vi "test TCX read (installed 71).vi"() -> ()   [LabVIEW 2011] (continued)
xmlns=\"http://www.garmin.com/xmlschemas/ActivityExtension/v2\"><Watts>107</Watts></TPX></Extensions></Trackpoint><Trackpoint><Time>2008-03-03T14:04:57Z</Time><Position><LatitudeDegrees>35.860918</LatitudeDegrees><LongitudeDegrees>-78.895742</LongitudeDegrees></Position><AltitudeMeters>90.021</AltitudeMeters><DistanceMeters>8842.457</DistanceMeters><Cadence>0</Cadence></Trackpoint><Trackpoint><Time>2008-03-03T14:04:58Z</Time><Position><LatitudeDegrees>35.860915</LatitudeDegrees><LongitudeDegrees>-78.895606</LongitudeDegrees></Position><AltitudeMeters>90.021</AltitudeMeters><DistanceMeters>8854.741</DistanceMeters><Cadence>0</Cadence></Trackpoint><Trackpoint><Time>2008-03-03T14:04:59Z</Time><Position><LatitudeDegrees>35.860920</LatitudeDegrees><LongitudeDegrees>-78.895468</LongitudeDegrees></Position><AltitudeMeters>89.059</AltitudeMeters><DistanceMeters>8867.175</DistanceMeters><Cadence>0</Cadence></Trackpoint><Trackpoint><Time>2008-03-03T14:05:00Z</Time><Position><LatitudeDegrees>35.860930</LatitudeDegrees><LongitudeDegrees>-78.895327</LongitudeDegrees></Position><AltitudeMeters>87.617</AltitudeMeters><DistanceMeters>8879.941</DistanceMeters><Cadence>0</Cadence></Trackpoint><Trackpoint><Time>2008-03-03T14:05:01Z</Time><Position><LatitudeDegrees>35.860938</LatitudeDegrees><LongitudeDegrees>-78.895183</LongitudeDegrees></Position><AltitudeMeters>87.137</AltitudeMeters><DistanceMeters>8893.053</DistanceMeters><Cadence>0</Cadence></Trackpoint><Trackpoint><Time>2008-03-03T14:05:02Z</Time><Position><LatitudeDegrees>35.860939</LatitudeDegrees><LongitudeDegrees>-78.895036</LongitudeDegrees></Position><AltitudeMeters>86.656</AltitudeMeters><DistanceMeters>8906.286</DistanceMeters><Cadence>0</Cadence></Trackpoint><Trackpoint><Time>2008-03-03T14:05:03Z</Time><Position><LatitudeDegrees>35.860942</LatitudeDegrees><LongitudeDegrees>-78.894890</LongitudeDegrees></Position><AltitudeMeters>85.695</AltitudeMeters><DistanceMeters>8919.586</DistanceMeters><Cadence>0</Cadence></Trackpoint><Trackpoint><Time>2008-03-03T14:05:04Z</Time><Position><LatitudeDegrees>35.860938</LatitudeDegrees><LongitudeDegrees>-78.894740</LongitudeDegrees></Position><AltitudeMeters>85.214</AltitudeMeters><DistanceMeters>8933.086</DistanceMeters><Cadence>0</Cadence></Trackpoint><Trackpoint><Time>2008-03-03T14:05:05Z</Time><Position><LatitudeDegrees>35.860924</LatitudeDegrees><LongitudeDegrees>-78.894592</LongitudeDegrees></Position><AltitudeMeters>84.253</AltitudeMeters><DistanceMeters>8946.535</DistanceMeters><Cadence>0</Cadence></Trackpoint><Trackpoint><Time>2008-03-03T14:05:06Z</Time><Position><LatitudeDegrees>35.860898</LatitudeDegrees><LongitudeDegrees>-78.894446</LongitudeDegrees></Position><AltitudeMeters>83.291</AltitudeMeters><DistanceMeters>8959.948</DistanceMeters><Cadence>0</Cadence></Trackpoint><Trackpoint><Time>2008-03-03T14:05:07Z</Time><Position><LatitudeDegrees>35.860875</LatitudeDegrees><LongitudeDegrees>-78.894304</LongitudeDegrees></Position><AltitudeMeters>83.772</AltitudeMeters><DistanceMeters>8973.048</DistanceMeters><Cadence>0</Cadence></Trackpoint><Trackpoint><Time>2008-03-03T14:05:08Z</Time><Position><LatitudeDegrees>35.860851</LatitudeDegrees><LongitudeDegrees>-78.894163</LongitudeDegrees></Position><AltitudeMeters>82.811</AltitudeMeters><DistanceMeters>8985.948</DistanceMeters><Cadence>0</Cadence></Trackpoint><Trackpoint><Time>2008-03-03T14:05:09Z</Time><Position><LatitudeDegrees>35.860831</LatitudeDegrees><LongitudeDegrees>-78.894026</LongitudeDegrees></Position><AltitudeMeters>82.330</AltitudeMeters><DistanceMeters>8998.589</DistanceMeters><Cadence>0</Cadence></Trackpoint><Trackpoint><Time>2008-03-03T14:05:10Z</Time><Position><LatitudeDegrees>35.860809</LatitudeDegrees><LongitudeDegrees>-78.893890</LongitudeDegrees></Position><AltitudeMeters>81.849</AltitudeMeters><DistanceMeters>9011.048</DistanceMeters><Cadence>4</Cadence><Extensions><TPX xmlns=\"http://www.garmin.com/xmlschemas/ActivityExtension/v2\"><Watts>0</Watts></TPX></Extensions></Trackpoint><Trackpoint><Time>2008-03-03T14:05:11Z</Time><Position><LatitudeDegrees>35.860788</LatitudeDegrees><LongitudeDegrees>-78.893758</LongitudeDegrees></Position><AltitudeMeters>81.849</AltitudeMeters><DistanceMeters>9023.194</DistanceMeters><Cadence>4</Cadence><Extensions><TPX xmlns=\"http://www.garmin.com/xmlschemas/ActivityExtension/v2\"><Watts>0</Watts></TPX></Extensions></Trackpoint><Trackpoint><Time>2008-03-03T14:05:12Z</Time><Position><LatitudeDegrees>35.860769</LatitudeDegrees><LongitudeDegrees>-78.893628</LongitudeDegrees></Position><AltitudeMeters>81.369</AltitudeMeters><DistanceMeters>9035.092</DistanceMeters><Cadence>71</Cadence><Extensions><TPX xmlns=\"http://www.garmin.com/xmlschemas/ActivityExtension/v2\"><Watts>90</Watts></TPX></Extensions></Trackpoint><Trackpoint><Time>2008-03-03T14:05:13Z</Time><Position><LatitudeDegrees>35.860753</LatitudeDegrees><LongitudeDegrees>-78.893502</LongitudeDegrees></Position><AltitudeMeters>81.849</AltitudeMeters><DistanceMeters>9046.647</DistanceMeters><Cadence>84</Cadence><Extensions><TPX xmlns=\"http://www.garmin.com/xmlschemas/ActivityExtension/v2\"><Watts>145</Watts></TPX></Extensions></Trackpoint><Trackpoint><Time>2008-03-03T14:05:14Z</Time><Position><LatitudeDegrees>35.860738</LatitudeDegrees><LongitudeDegrees>-78.893381</LongitudeDegrees></Position><AltitudeMeters>81.849</AltitudeMeters><DistanceMeters>9057.588</DistanceMeters><Cadence>81</Cadence><Extensions><TPX xmlns=\"http://www.garmin.com/xmlschemas/ActivityExtension/v2\"><Watts>197</Watts></TPX></Extensions></Trackpoint><Trackpoint><Time>2008-03-03T14:05:15Z</Time><Position><LatitudeDegrees>35.860725</LatitudeDegrees><LongitudeDegrees>-78.893268</LongitudeDegrees></Position><AltitudeMeters>82.811</AltitudeMeters><DistanceMeters>9067.873</DistanceMeters><Cadence>80</Cadence><Extensions><TPX xmlns=\"http://www.garmin.com/xmlschemas/ActivityExtension/v2\"><Watts>211</Watts></TPX></Extensions></Trackpoint><Trackpoint><Time>2008-03-03T14:05:16Z</Time><Position><LatitudeDegrees>35.860714</LatitudeDegrees><LongitudeDegrees>-78.893164</LongitudeDegrees></Position><AltitudeMeters>83.291</AltitudeMeters><DistanceMeters>9077.331</DistanceMeters><Cadence>78</Cadence><Extensions><TPX xmlns=\"http://www.garmin.com/xmlschemas/ActivityExtension/v2\"><Watts>233</Watts></TPX></Extensions></Trackpoint><Trackpoint><Time>2008-03-03T14:05:17Z</Time><Position><LatitudeDegrees>35.860703</LatitudeDegrees><LongitudeDegrees>-78.893065</LongitudeDegrees></Position><AltitudeMeters>84.253</AltitudeMeters><DistanceMeters>9086.308</DistanceMeters><Cadence>73</Cadence><Extensions><TPX xmlns=\"http://www.garmin.com/xmlschemas/ActivityExtension/v2\"><Watts>281</Watts></TPX></Extensions></Trackpoint><Trackpoint><Time>2008-03-03T14:05:18Z</Time><Position><LatitudeDegrees>35.860691</LatitudeDegrees><LongitudeDegrees>-78.892970</LongitudeDegrees></Position><AltitudeMeters>84.253</AltitudeMeters><DistanceMeters>9095.026</DistanceMeters><Cadence>73</Cadence><Extensions><TPX xmlns=\"http://www.garmin.com/xmlschemas/ActivityExtension/v2\"><Watts>281</Watts></TPX></Extensions></Trackpoint><Trackpoint><Time>2008-03-03T14:05:19Z</Time><Position><LatitudeDegrees>35.860678</LatitudeDegrees><LongitudeDegrees>-78.892875</LongitudeDegrees></Position><AltitudeMeters>84.733</AltitudeMeters><DistanceMeters>9103.671</DistanceMeters><Cadence>72</Cadence><Extensions><TPX xmlns=\"http://www.garmin.com/xmlschemas/ActivityExtension/v2\"><Watts>458</Watts></TPX></Extensions></Trackpoint><Trackpoint><Time>2008-03-03T14:05:20Z</Time><Position><LatitudeDegrees>35.860666</LatitudeDegrees><LongitudeDegrees>-78.892780</LongitudeDegrees></Position><AltitudeMeters>84.733</AltitudeMeters><DistanceMeters>9112.350</DistanceMeters><Cadence>72</Cadence><Extensions><TPX xmlns=\"http://www.garmin.com/xmlschemas/ActivityExtension/v2\"><Watts>588</Watts></TPX></Extensions></Trackpoint><Trackpoint><Time>2008-03-03T14:05:21Z</Time><Position><LatitudeDegrees>35.860655</LatitudeDegrees><LongitudeDegrees>-78.892685</LongitudeDegrees></Position><AltitudeMeters>85.214</AltitudeMeters><DistanceMeters>9121.041</DistanceMeters><Cadence>72</Cadence><Extensions><TPX xmlns=\"http://www.garmin.com/xmlschemas/ActivityExtension/v2\"><Watts>591</Watts></TPX></Extensions></Trackpoint><Trackpoint><Time>2008-03-03T14:05:22Z</Time><Position><LatitudeDegrees>35.860642</LatitudeDegrees><LongitudeDegrees>-78.892589</LongitudeDegrees></Position><AltitudeMeters>85.214</AltitudeMeters><DistanceMeters>9129.810</DistanceMeters><Cadence>72</Cadence><Extensions><TPX xmlns=\"http://www.garmin.com/xmlschemas/ActivityExtension/v2\"><Watts>493</Watts></TPX></Extensions></Trackpoint><Trackpoint><Time>2008-03-03T14:05:23Z</Time><Position><LatitudeDegrees>35.860628</LatitudeDegrees><LongitudeDegrees>-78.892493</LongitudeDegrees></Position><AltitudeMeters>85.695</AltitudeMeters><DistanceMeters>9138.619</DistanceMeters><Cadence>72</Cadence><Extensions><TPX xmlns=\"http://www.garmin.com/xmlschemas/ActivityExtension/v2\"><Watts>472</Watts></TPX></Extensions></Trackpoint><Trackpoint><Time>2008-03-03T14:05:24Z</Time><Position><LatitudeDegrees>35.860618</LatitudeDegrees><LongitudeDegrees>-78.892396</LongitudeDegrees></Position><AltitudeMeters>86.175</AltitudeMeters><DistanceMeters>9147.436</DistanceMeters><Cadence>73</Cadence><Extensions><TPX xmlns=\"http://www.garmin.com/xmlschemas/ActivityExtension/v2\"><Watts>438</Watts></TPX></Extensions></Trackpoint><Trackpoint><Time>2008-03-03T14:05:25Z</Time><Position><LatitudeDegrees>35.860608</LatitudeDegrees><LongitudeDegrees>-78.892296</LongitudeDegrees></Position><AltitudeMeters>85.695</AltitudeMeters><DistanceMeters>9156.547</DistanceMeters><Cadence>74</Cadence><Extensions><TPX xmlns=\"http://www.garmin.com/xmlschemas/ActivityExtension/v2\"><Watts>433</Watts></TPX></Extensions></Trackpoint><Trackpoint><Time>2008-03-03T14:05:26Z</Time><Position><LatitudeDegrees>35.860601</LatitudeDegrees><LongitudeDegrees>-78.892192</LongitudeDegrees></Position><AltitudeMeters>86.175</AltitudeMeters><DistanceMeters>9165.991</DistanceMeters><Cadence>76</Cadence><Extensions><TPX xmlns=\"http://www.garmin.com/xmlschemas/ActivityExtension/v2\"><Watts>430</Watts></TPX></Extensions></Trackpoint><Trackpoint><Time>2008-03-03T14:05:27Z</Time><Position><LatitudeDegrees>35.860591</LatitudeDegrees><LongitudeDegrees>-78.892087</LongitudeDegrees></Position><AltitudeMeters>86.656</AltitudeMeters><DistanceMeters>9175.522</DistanceMeters><Cadence>80</Cadence><Extensions><TPX xmlns=\"http://www.garmin.com/xmlschemas/ActivityExtension/v2\"><Watts>528</Watts></TPX></Extensions></Trackpoint><Trackpoint><Time>2008-03-03T14:05:28Z</Time><Position><LatitudeDegrees>35.860585</LatitudeDegrees><LongitudeDegrees>-78.891979</LongitudeDegrees></Position><AltitudeMeters>86.175</AltitudeMeters><DistanceMeters>9185.361</DistanceMeters><Cadence>81</Cadence><Extensions><TPX xmlns=\"http://www.garmin.com/xmlschemas/ActivityExtension/v2\"><Watts>536</Watts></TPX></Extensions></Trackpoint><Trackpoint><Time>2008-03-03T14:05:29Z</Time><Position><LatitudeDegrees>35.860574</LatitudeDegrees><LongitudeDegrees>-78.891869</LongitudeDegrees></Position><AltitudeMeters>87.137</AltitudeMeters><DistanceMeters>9195.392</DistanceMeters><Cadence>82</Cadence><Extensions><TPX xmlns=\"http://www.garmin.com/xmlschemas/ActivityExtension/v2\"><Watts>542</Watts></TPX></Extensions></Trackpoint><Trackpoint><Time>2008-03-03T14:05:30Z</Time><Position><LatitudeDegrees>35.860564</LatitudeDegrees><LongitudeDegrees>-78.891759</LongitudeDegrees></Position><AltitudeMeters>87.137</AltitudeMeters><DistanceMeters>9205.390</DistanceMeters><Cadence>82</Cadence><Extensions><TPX xmlns=\"http://www.garmin.com/xmlschemas/ActivityExtension/v2\"><Watts>523</Watts></TPX></Extensions></Trackpoint><Trackpoint><Time>2008-03-03T14:05:31Z</Time><Position><LatitudeDegrees>35.860551</LatitudeDegrees><LongitudeDegrees>-78.891649</LongitudeDegrees></Position><AltitudeMeters>87.617</AltitudeMeters><DistanceMeters>9215.414</DistanceMeters><Cadence>86</Cadence><Extensions><TPX xmlns=\"http://www.garmin.com/xmlschemas/ActivityExtension/v2\"><Watts>515</Watts></TPX></Extensions></Trackpoint><Trackpoint><Time>2008-03-03T14:05:32Z</Time><Position><LatitudeDegrees>35.860540</LatitudeDegrees><LongitudeDegrees>-78.891537</LongitudeDegrees></Position><AltitudeMeters>87.617</AltitudeMeters><DistanceMeters>9225.561</DistanceMeters><Cadence>82</Cadence><Extensions><TPX xmlns=\"http://www.garmin.com/xmlschemas/ActivityExtension/v2\"><Watts>495</Watts></TPX></Extensions></Trackpoint><Trackpoint><Time>2008-03-03T14:05:33Z</Time><Position><LatitudeDegrees>35.860528</LatitudeDegrees><LongitudeDegrees>-78.891428</LongitudeDegrees></Position><AltitudeMeters>87.617</AltitudeMeters><DistanceMeters>9235.504</DistanceMeters><Cadence>80</Cadence><Extensions><TPX xmlns=\"http://www.garmin.com/xmlschemas/ActivityExtension/v2\"><Watts>168</Watts></TPX></Extensions></Trackpoint><Trackpoint><Time>2008-03-03T14:05:34Z</Time><Position><LatitudeDegrees>35.860516</LatitudeDegrees><LongitudeDegrees>-78.891323</LongitudeDegrees></Position><AltitudeMeters>87.617</AltitudeMeters><DistanceMeters>9245.120</DistanceMeters><Cadence>78</Cadence><Extensions><TPX xmlns=\"http://www.garmin.com/xmlschemas/ActivityExtension/v2\"><Watts>157</Watts></TPX></Extensions></Trackpoint><Trackpoint><Time>2008-03-03T14:05:35Z</Time><Position><LatitudeDegrees>35.860506</LatitudeDegrees><LongitudeDegrees>-78.891219</LongitudeDegrees></Position><AltitudeMeters>87.617</AltitudeMeters><DistanceMeters>9254.466</DistanceMeters><Cadence>76</Cadence><Extensions><TPX xmlns=\"http://www.garmin.com/xmlschemas/ActivityExtension/v2\"><Watts>146</Watts></TPX></Extensions></Trackpoint><Trackpoint><Time>2008-03-03T14:05:36Z</Time><Position><LatitudeDegrees>35.860495</LatitudeDegrees><LongitudeDegrees>-78.891119</LongitudeDegrees></Position><AltitudeMeters>87.617</AltitudeMeters><DistanceMeters>9263.595</DistanceMeters><Cadence>75</Cadence><Extensions><TPX xmlns=\"http://www.garmin.com/xmlschemas/ActivityExtension/v2\"><Watts>141</Watts></TPX></Extensions></Trackpoint><Trackpoint><Time>2008-03-03T14:05:37Z</Time><Position><LatitudeDegrees>35.860483</LatitudeDegrees><LongitudeDegrees>-78.891021</LongitudeDegrees></Position><AltitudeMeters>87.617</AltitudeMeters><DistanceMeters>9272.575</DistanceMeters><Cadence>73</Cadence><Extensions><TPX xmlns=\"http://www.garmin.com/xmlschemas/ActivityExtension/v2\"><Watts>139</Watts></TPX></Extensions></Trackpoint><Trackpoint><Time>2008-03-03T14:05:38Z</Time><Position><LatitudeDegrees>35.860470</LatitudeDegrees><LongitudeDegrees>-78.890924</LongitudeDegrees></Position><AltitudeMeters>87.617</AltitudeMeters><DistanceMeters>9281.458</DistanceMeters><Cadence>72</Cadence><Extensions><TPX xmlns=\"http://www.garmin.com/xmlschemas/ActivityExtension/v2\"><Watts>141</Watts></TPX></Extensions></Trackpoint><Trackpoint><Time>2008-03-03T14:05:39Z</Time><Position><LatitudeDegrees>35.860457</LatitudeDegrees><LongitudeDegrees>-78.890829</LongitudeDegrees></Position><AltitudeMeters>88.098</AltitudeMeters><DistanceMeters>9290.096</DistanceMeters><Cadence>71</Cadence><Extensions><TPX xmlns=\"http://www.garmin.com/xmlschemas/ActivityExtension/v2\"><Watts>141</Watts></TPX></Extensions></Trackpoint><Trackpoint><Time>2008-03-03T14:05:40Z</Time><Position><LatitudeDegrees>35.860444</LatitudeDegrees><LongitudeDegrees>-78.890736</LongitudeDegrees></Position><AltitudeMeters>88.098</AltitudeMeters><DistanceMeters>9298.659</DistanceMeters><Cadence>71</Cadence><Extensions><TPX xmlns=\"http://www.garmin.com/xmlschemas/ActivityExtension/v2\"><Watts>140</Watts></TPX></Extensions></Trackpoint><Trackpoint><Time>2008-03-03T14:05:41Z</Time><Position><LatitudeDegrees>35.860431</LatitudeDegrees><LongitudeDegrees>-78.890644</LongitudeDegrees></Position><AltitudeMeters>88.098</AltitudeMeters><DistanceMeters>9307.081</DistanceMeters><Cadence>70</Cadence><Extensions><TPX xmlns=\"http://www.garmin.com/xmlschemas/ActivityExtension/v2\"><Watts>150</Watts></TPX></Extensions></Trackpoint><Trackpoint><Time>2008-03-03T14:05:42Z</Time><Position><LatitudeDegrees>35.860420</LatitudeDegrees><LongitudeDegrees>-78.890553</LongitudeDegrees></Position><AltitudeMeters>88.098</AltitudeMeters><DistanceMeters>9315.363</DistanceMeters><Cadence>74</Cadence><Extensions><TPX xmlns=\"http://www.garmin.com/xmlschemas/ActivityExtension/v2\"><Watts>141</Watts></TPX></Extensions></Trackpoint><Trackpoint><Time>2008-03-03T14:05:43Z</Time><Position><LatitudeDegrees>35.860407</LatitudeDegrees><LongitudeDegrees>-78.890463</LongitudeDegrees></Position><AltitudeMeters>88.579</AltitudeMeters><DistanceMeters>9323.592</DistanceMeters><Cadence>76</Cadence><Extensions><TPX xmlns=\"http://www.garmin.com/xmlschemas/ActivityExtension/v2\"><Watts>133</Watts></TPX></Extensions></Trackpoint><Trackpoint><Time>2008-03-03T14:05:44Z</Time><Position><LatitudeDegrees>35.860393</LatitudeDegrees><LongitudeDegrees>-78.890375</LongitudeDegrees></Position><AltitudeMeters>88.579</AltitudeMeters><DistanceMeters>9331.684</DistanceMeters><Cadence>75</Cadence><Extensions><TPX xmlns=\"http://www.garmin.com/xmlschemas/ActivityExtension/v2\"><Watts>171</Watts></TPX></Extensions></Trackpoint><Trackpoint><Time>2008-03-03T14:05:45Z</Time><Position><LatitudeDegrees>35.860381</LatitudeDegrees><LongitudeDegrees>-78.890287</LongitudeDegrees></Position><AltitudeMeters>89.059</AltitudeMeters><DistanceMeters>9339.685</DistanceMeters><Cadence>75</Cadence><Extensions><TPX xmlns=\"http://www.garmin.com/xmlschemas/ActivityExtension/v2\"><Watts>207</Watts></TPX></Extensions></Trackpoint><Trackpoint><Time>2008-03-03T14:05:46Z</Time><Position><LatitudeDegrees>35.860372</LatitudeDegrees><LongitudeDegrees>-78.890200</LongitudeDegrees></Position><AltitudeMeters>88.579</AltitudeMeters><DistanceMeters>9347.658</DistanceMeters><Cadence>74</Cadence><Extensions><TPX xmlns=\"http://www.garmin.com/xmlschemas/ActivityExtension/v2\"><Watts>227</Watts></TPX></Extensions></Trackpoint><Trackpoint><Time>2008-03-03T14:05:47Z</Time><Position><LatitudeDegrees>35.860362</LatitudeDegrees><LongitudeDegrees>-78.890113</LongitudeDegrees></Position><AltitudeMeters>89.059</AltitudeMeters><DistanceMeters>9355.555</DistanceMeters><Cadence>73</Cadence><Extensions><TPX xmlns=\"http://www.garmin.com/xmlschemas/ActivityExtension/v2\"><Watts>228</Watts></TPX></Extensions></Trackpoint><Trackpoint><Time>2008-03-03T14:05:48Z</Time><Position><LatitudeDegrees>35.860352</LatitudeDegrees><LongitudeDegrees>-78.890027</LongitudeDegrees></Position><AltitudeMeters>89.540</AltitudeMeters><DistanceMeters>9363.416</DistanceMeters><Cadence>73</Cadence><Extensions><TPX xmlns=\"http://www.garmin.com/xmlschemas/ActivityExtension/v2\"><Watts>231</Watts></TPX></Extensions></Trackpoint><Trackpoint><Time>2008-03-03T14:05:49Z</Time><Position><LatitudeDegrees>35.860343</LatitudeDegrees><LongitudeDegrees>-78.889942</LongitudeDegrees></Position><AltitudeMeters>89.540</AltitudeMeters><DistanceMeters>9371.137</DistanceMeters><Cadence>72</Cadence><Extensions><TPX xmlns=\"http://www.garmin.com/xmlschemas/ActivityExtension/v2\"><Watts>246</Watts></TPX></Extensions></Trackpoint><Trackpoint><Time>2008-03-03T14:05:50Z</Time><Position><LatitudeDegrees>35.860334</LatitudeDegrees><LongitudeDegrees>-78.889859</LongitudeDegrees></Position><AltitudeMeters>90.021</AltitudeMeters><DistanceMeters>9378.760</DistanceMeters><Cadence>72</Cadence><Extensions><TPX xmlns=\"http://www.garmin.com/xmlschemas/ActivityExtension/v2\"><Watts>246</Watts></TPX></Extensions></Trackpoint><Trackpoint><Time>2008-03-03T14:05:51Z</Time><Position><LatitudeDegrees>35.860323</LatitudeDegrees><LongitudeDegrees>-78.889776</LongitudeDegrees></Position><AltitudeMeters>90.021</AltitudeMeters><DistanceMeters>9386.328</DistanceMeters><Cadence>70</Cadence><Extensions><TPX xmlns=\"http://www.garmin.com/xmlschemas/ActivityExtension/v2\"><Watts>306</Watts></TPX></Extensions></Trackpoint><Trackpoint><Time>2008-03-03T14:05:52Z</Time><Position><LatitudeDegrees>35.860313</LatitudeDegrees><LongitudeDegrees>-78.889694</LongitudeDegrees></Position><AltitudeMeters>90.501</AltitudeMeters><DistanceMeters>9393.784</DistanceMeters><Cadence>70</Cadence><Extensions><TPX xmlns=\"http://www.garmin.com/xmlschemas/ActivityExtension/v2\"><Watts>305</Watts></TPX></Extensions></Trackpoint><Trackpoint><Time>2008-03-03T14:05:53Z</Time><Position><LatitudeDegrees>35.860303</LatitudeDegrees><LongitudeDegrees>-78.889613</LongitudeDegrees></Position><AltitudeMeters>90.982</AltitudeMeters><DistanceMeters>9401.264</DistanceMeters><Cadence>69</Cadence><Extensions><TPX xmlns=\"http://www.garmin.com/xmlschemas/ActivityExtension/v2\"><Watts>334</Watts></TPX></Extensions></Trackpoint><Trackpoint><Time>2008-03-03T14:05:54Z</Time><Position><LatitudeDegrees>35.860294</LatitudeDegrees><LongitudeDegrees>-78.889530</LongitudeDegrees></Position><AltitudeMeters>91.463</AltitudeMeters><DistanceMeters>9408.714</DistanceMeters><Cadence>70</Cadence><Extensions><TPX xmlns=\"http://www.garmin.com/xmlschemas/ActivityExtension/v2\"><Watts>368</Watts></TPX></Extensions></Trackpoint><Trackpoint><Time>2008-03-03T14:05:55Z</Time><Position><LatitudeDegrees>35.860285</LatitudeDegrees><LongitudeDegrees>-78.889448</LongitudeDegrees></Position><AltitudeMeters>91.463</AltitudeMeters><DistanceMeters>9416.229</DistanceMeters><Cadence>70</Cadence><Extensions><TPX xmlns=\"http://www.garmin.com/xmlschemas/ActivityExtension/v2\"><Watts>382</Watts></TPX></Extensions></Trackpoint><Trackpoint><Time>2008-03-03T14:05:56Z</Time><Position><LatitudeDegrees>35.860275</LatitudeDegrees><LongitudeDegrees>-78.889366</LongitudeDegrees></Position><AltitudeMeters>91.463</AltitudeMeters><DistanceMeters>9423.748</DistanceMeters><Cadence>70</Cadence><Extensions><TPX xmlns=\"http://www.garmin.com/xmlschemas/ActivityExtension/v2\"><Watts>382</Watts></TPX></Extensions></Trackpoint><Trackpoint><Time>2008-03-03T14:05:57Z</Time><Position><LatitudeDegrees>35.860264</LatitudeDegrees><LongitudeDegrees>-78.889285</LongitudeDegrees></Position><AltitudeMeters>91.943</AltitudeMeters><DistanceMeters>9431.158</DistanceMeters><Cadence>70</Cadence><Extensions><TPX xmlns=\"http://www.garmin.com/xmlschemas/ActivityExtension/v2\"><Watts>383</Watts></TPX></Extensions></Trackpoint><Trackpoint><Time>2008-03-03T14:05:58Z</Time><Position><LatitudeDegrees>35.860254</LatitudeDegrees><LongitudeDegrees>-78.889204</LongitudeDegrees></Position><AltitudeMeters>92.424</AltitudeMeters><DistanceMeters>9438.506</DistanceMeters><Cadence>68</Cadence><Extensions><TPX xmlns=\"http://www.garmin.com/xmlschemas/ActivityExtension/v2\"><Watts>337</Watts></TPX></Extensions></Trackpoint><Trackpoint><Time>2008-03-03T14:05:59Z</Time><Position><LatitudeDegrees>35.860243</LatitudeDegrees><LongitudeDegrees>-78.889125</LongitudeDegrees></Position><AltitudeMeters>92.424</AltitudeMeters><DistanceMeters>9445.806</DistanceMeters><Cadence>67</Cadence><Extensions><TPX xmlns=\"http://www.garmin.com/xmlschemas/ActivityExtension/v2\"><Watts>322</Watts></TPX></Extensions></Trackpoint><Trackpoint><Time>2008-03-03T14:06:00Z</Time><Position><LatitudeDegrees>35.860232</LatitudeDegrees><LongitudeDegrees>-78.889046</LongitudeDegrees></Position><AltitudeMeters>92.905</AltitudeMeters><DistanceMeters>9453.028</DistanceMeters><Cadence>67</Cadence><Extensions><TPX xmlns=\"http://www.garmin.com/xmlschemas/ActivityExtension/v2\"><Watts>324</Watts></TPX></Extensions></Trackpoint><Trackpoint><Time>2008-03-03T14:06:01Z</Time><Position><LatitudeDegrees>35.860219</LatitudeDegrees><LongitudeDegrees>-78.888967</LongitudeDegrees></Position><AltitudeMeters>92.905</AltitudeMeters><DistanceMeters>9460.292</DistanceMeters><Cadence>67</Cadence><Extensions><TPX xmlns=\"http://www.garmin.com/xmlschemas/ActivityExtension/v2\"><Watts>317</Watts></TPX></Extensions></Trackpoint><Trackpoint><Time>2008-03-03T14:06:02Z</Time><Position><LatitudeDegrees>35.860209</LatitudeDegrees><LongitudeDegrees>-78.888888</LongitudeDegrees></Position><AltitudeMeters>92.905</AltitudeMeters><DistanceMeters>9467.478</DistanceMeters><Cadence>67</Cadence><Extensions><TPX xmlns=\"http://www.garmin.com/xmlschemas/ActivityExtension/v2\"><Watts>317</Watts></TPX></Extensions></Trackpoint><Trackpoint><Time>2008-03-03T14:06:03Z</Time><Position><LatitudeDegrees>35.860199</LatitudeDegrees><LongitudeDegrees>-78.888810</LongitudeDegrees></Position><AltitudeMeters>93.385</AltitudeMeters><DistanceMeters>9474.705</DistanceMeters><Cadence>67</Cadence><Extensions><TPX xmlns=\"http://www.garmin.com/xmlschemas/ActivityExtension/v2\"><Watts>312</Watts></TPX></Extensions></Trackpoint><Trackpoint><Time>2008-03-03T14:06:04Z</Time><Position><LatitudeDegrees>35.860190</LatitudeDegrees><LongitudeDegrees>-78.888731</LongitudeDegrees></Position><AltitudeMeters>93.866</AltitudeMeters><DistanceMeters>9481.862</DistanceMeters><Cadence>67</Cadence><Extensions><TPX xmlns=\"http://www.garmin.com/xmlschemas/ActivityExtension/v2\"><Watts>294</Watts></TPX></Extensions></Trackpoint><Trackpoint><Time>2008-03-03T14:06:05Z</Time><Position><LatitudeDegrees>35.860177</LatitudeDegrees><LongitudeDegrees>-78.888653</LongitudeDegrees></Position><AltitudeMeters>93.866</AltitudeMeters><DistanceMeters>9489.069</DistanceMeters><Cadence>67</Cadence><Extensions><TPX xmlns=\"http://www.garmin.com/xmlschemas/ActivityExtension/v2\"><Watts>283</Watts></TPX></Extensions></Trackpoint><Trackpoint><Time>2008-03-03T14:06:06Z</Time><Position><LatitudeDegrees>35.860163</LatitudeDegrees><LongitudeDegrees>-78.888574</LongitudeDegrees></Position><AltitudeMeters>93.866</AltitudeMeters><DistanceMeters>9496.394</DistanceMeters><Cadence>68</Cadence><Extensions><TPX xmlns=\"http://www.garmin.com/xmlschemas/ActivityExtension/v2\"><Watts>257</Watts></TPX></Extensions></Trackpoint><Trackpoint><Time>2008-03-03T14:06:07Z</Time><Position><LatitudeDegrees>35.860149</LatitudeDegrees><LongitudeDegrees>-78.888494</LongitudeDegrees></Position><AltitudeMeters>94.347</AltitudeMeters><DistanceMeters>9503.709</DistanceMeters><Cadence>68</Cadence><Extensions><TPX xmlns=\"http://www.garmin.com/xmlschemas/ActivityExtension/v2\"><Watts>260</Watts></TPX></Extensions></Trackpoint><Trackpoint><Time>2008-03-03T14:06:08Z</Time><Position><LatitudeDegrees>35.860137</LatitudeDegrees><LongitudeDegrees>-78.888413</LongitudeDegrees></Position><AltitudeMeters>94.347</AltitudeMeters><DistanceMeters>9511.131</DistanceMeters><Cadence>69</Cadence><Extensions><TPX xmlns=\"http://www.garmin.com/xmlschemas/ActivityExtension/v2\"><Watts>231</Watts></TPX></Extensions></Trackpoint><Trackpoint><Time>2008-03-03T14:06:09Z</Time><Position><LatitudeDegrees>35.860126</LatitudeDegrees><LongitudeDegrees>-78.888332</LongitudeDegrees></Position><AltitudeMeters>94.347</AltitudeMeters><DistanceMeters>9518.592</DistanceMeters><Cadence>69</Cadence><Extensions><TPX xmlns=\"http://www.garmin.com/xmlschemas/ActivityExtension/v2\"><Watts>230</Watts></TPX></Extensions></Trackpoint><Trackpoint><Time>2008-03-03T14:06:10Z</Time><Position><LatitudeDegrees>35.860114</LatitudeDegrees><LongitudeDegrees>-78.888250</LongitudeDegrees></Position><AltitudeMeters>94.827</AltitudeMeters><DistanceMeters>9526.155</DistanceMeters><Cadence>70</Cadence><Extensions><TPX xmlns=\"http://www.garmin.com/xmlschemas/ActivityExtension/v2\"><Watts>219</Watts></TPX></Extensions></Trackpoint><Trackpoint><Time>2008-03-03T14:06:11Z</Time><Position><LatitudeDegrees>35.860102</LatitudeDegrees><LongitudeDegrees>-78.888167</LongitudeDegrees></Position><AltitudeMeters>94.347</AltitudeMeters><DistanceMeters>9533.737</DistanceMeters><Cadence>70</Cadence><Extensions><TPX xmlns=\"http://www.garmin.com/xmlschemas/ActivityExtension/v2\"><Watts>191</Watts></TPX></Extensions></Trackpoint><Trackpoint><Time>2008-03-03T14:06:12Z</Time><Position><LatitudeDegrees>35.860089</LatitudeDegrees><LongitudeDegrees>-78.888084</LongitudeDegrees></Position><AltitudeMeters>94.827</AltitudeMeters><DistanceMeters>9541.394</DistanceMeters><Cadence>71</Cadence><Extensions><TPX xmlns=\"http://www.garmin.com/xmlschemas/ActivityExtension/v2\"><Watts>166</Watts></TPX></Extensions></Trackpoint><Trackpoint><Time>2008-03-03T14:06:13Z</Time><Position><LatitudeDegrees>35.860076</LatitudeDegrees><LongitudeDegrees>-78.887999</LongitudeDegrees></Position><AltitudeMeters>94.347</AltitudeMeters><DistanceMeters>9549.201</DistanceMeters><Cadence>72</Cadence><Extensions><TPX xmlns=\"http://www.garmin.com/xmlschemas/ActivityExtension/v2\"><Watts>157</Watts></TPX></Extensions></Trackpoint><Trackpoint><Time>2008-03-03T14:06:14Z</Time><Position><LatitudeDegrees>35.860064</LatitudeDegrees><LongitudeDegrees>-78.887913</LongitudeDegrees></Position><AltitudeMeters>94.347</AltitudeMeters><DistanceMeters>9557.050</DistanceMeters><Cadence>73</Cadence><Extensions><TPX xmlns=\"http://www.garmin.com/xmlschemas/ActivityExtension/v2\"><Watts>151</Watts></TPX></Extensions></Trackpoint><Trackpoint><Time>2008-03-03T14:06:15Z</Time><Position><LatitudeDegrees>35.860051</LatitudeDegrees><LongitudeDegrees>-78.887826</LongitudeDegrees></Position><AltitudeMeters>94.347</AltitudeMeters><DistanceMeters>9565.059</DistanceMeters><Cadence>74</Cadence><Extensions><TPX xmlns=\"http://www.garmin.com/xmlschemas/ActivityExtension/v2\"><Watts>148</Watts></TPX></Extensions></Trackpoint><Trackpoint><Time>2008-03-03T14:06:16Z</Time><Position><LatitudeDegrees>35.860036</LatitudeDegrees><LongitudeDegrees>-78.887738</LongitudeDegrees></Position><AltitudeMeters>94.347</AltitudeMeters><DistanceMeters>9573.151</DistanceMeters><Cadence>76</Cadence><Extensions><TPX xmlns=\"http://www.garmin.com/xmlschemas/ActivityExtension/v2\"><Watts>144</Watts></TPX></Extensions></Trackpoint><Trackpoint><Time>2008-03-03T14:06:17Z</Time><Position><LatitudeDegrees>35.860023</LatitudeDegrees><LongitudeDegrees>-78.887649</LongitudeDegrees></Position><AltitudeMeters>94.347</AltitudeMeters><DistanceMeters>9581.350</DistanceMeters><Cadence>76</Cadence><Extensions><TPX xmlns=\"http://www.garmin.com/xmlschemas/ActivityExtension/v2\"><Watts>145</Watts></TPX></Extensions></Trackpoint><Trackpoint><Time>2008-03-03T14:06:18Z</Time><Position><LatitudeDegrees>35.860012</LatitudeDegrees><LongitudeDegrees>-78.887558</LongitudeDegrees></Position><AltitudeMeters>94.347</AltitudeMeters><DistanceMeters>9589.688</DistanceMeters><Cadence>78</Cadence><Extensions><TPX xmlns=\"http://www.garmin.com/xmlschemas/ActivityExtension/v2\"><Watts>112</Watts></TPX></Extensions></Trackpoint><Trackpoint><Time>2008-03-03T14:06:19Z</Time><Position><LatitudeDegrees>35.860003</LatitudeDegrees><LongitudeDegrees>-78.887465</LongitudeDegrees></Position><AltitudeMeters>94.347</AltitudeMeters><DistanceMeters>9598.128</DistanceMeters><Cadence>78</Cadence><Extensions><TPX xmlns=\"http://www.garmin.com/xmlschemas/ActivityExtension/v2\"><Watts>96</Watts></TPX></Extensions></Trackpoint><Trackpoint><Time>2008-03-03T14:06:20Z</Time><Position><LatitudeDegrees>35.859995</LatitudeDegrees><LongitudeDegrees>-78.887372</LongitudeDegrees></Position><AltitudeMeters>93.866</AltitudeMeters><DistanceMeters>9606.686</DistanceMeters><Cadence>79</Cadence><Extensions><TPX xmlns=\"http://www.garmin.com/xmlschemas/ActivityExtension/v2\"><Watts>98</Watts></TPX></Extensions></Trackpoint><Trackpoint><Time>2008-03-03T14:06:21Z</Time><Position><LatitudeDegrees>35.859988</LatitudeDegrees><LongitudeDegrees>-78.887278</LongitudeDegrees></Position><AltitudeMeters>94.347</AltitudeMeters><DistanceMeters>9615.188</DistanceMeters><Cadence>79</Cadence><Extensions><TPX xmlns=\"http://www.garmin.com/xmlschemas/ActivityExtension/v2\"><Watts>106</Watts></TPX></Extensions></Trackpoint><Trackpoint><Time>2008-03-03T14:06:22Z</Time><Position><LatitudeDegrees>35.859978</LatitudeDegrees><LongitudeDegrees>-78.887183</LongitudeDegrees></Position><AltitudeMeters>93.866</AltitudeMeters><DistanceMeters>9623.765</DistanceMeters><Cadence>79</Cadence><Extensions><TPX xmlns=\"http://www.garmin.com/xmlschemas/ActivityExtension/v2\"><Watts>114</Watts></TPX></Extensions></Trackpoint><Trackpoint><Time>2008-03-03T14:06:23Z</Time><Position><LatitudeDegrees>35.859967</LatitudeDegrees><LongitudeDegrees>-78.887090</LongitudeDegrees></Position><AltitudeMeters>93.866</AltitudeMeters><DistanceMeters>9632.330</DistanceMeters><Cadence>79</Cadence><Extensions><TPX xmlns=\"http://www.garmin.com/xmlschemas/ActivityExtension/v2\"><Watts>116</Watts></TPX></Extensions></Trackpoint><Trackpoint><Time>2008-03-03T14:06:24Z</Time><Position><LatitudeDegrees>35.859953</LatitudeDegrees><LongitudeDegrees>-78.886997</LongitudeDegrees></Position><AltitudeMeters>93.866</AltitudeMeters><DistanceMeters>9640.762</DistanceMeters><Cadence>78</Cadence><Extensions><TPX xmlns=\"http://www.garmin.com/xmlschemas/ActivityExtension/v2\"><Watts>105</Watts></TPX></Extensions></Trackpoint><Trackpoint><Time>2008-03-03T14:06:25Z</Time><Position><LatitudeDegrees>35.859937</LatitudeDegrees><LongitudeDegrees>-78.886907</LongitudeDegrees></Position><AltitudeMeters>93.866</AltitudeMeters><DistanceMeters>9649.090</DistanceMeters><Cadence>77</Cadence><Extensions><TPX xmlns=\"http://www.garmin.com/xmlschemas/ActivityExtension/v2\"><Watts>105</Watts></TPX></Extensions></Trackpoint><Trackpoint><Time>2008-03-03T14:06:26Z</Time><Position><LatitudeDegrees>35.859917</LatitudeDegrees><LongitudeDegrees>-78.886819</LongitudeDegrees></Position><AltitudeMeters>93.866</AltitudeMeters><DistanceMeters>9657.394</DistanceMeters><Cadence>76</Cadence><Extensions><TPX xmlns=\"http://www.garmin.com/xmlschemas/ActivityExtension/v2\"><Watts>126</Watts></TPX></Extensions></Trackpoint><Trackpoint><Time>2008-03-03T14:06:27Z</Time><Position><LatitudeDegrees>35.859897</LatitudeDegrees><LongitudeDegrees>-78.886731</LongitudeDegrees></Position><AltitudeMeters>93.866</AltitudeMeters><DistanceMeters>9665.654</DistanceMeters><Cadence>76</Cadence><Extensions><TPX xmlns=\"http://www.garmin.com/xmlschemas/ActivityExtension/v2\"><Watts>128</Watts></TPX></Extensions></Trackpoint><Trackpoint><Time>2008-03-03T14:06:28Z</Time><Position><LatitudeDegrees>35.859876</LatitudeDegrees><LongitudeDegrees>-78.886643</LongitudeDegrees></Position><AltitudeMeters>93.866</AltitudeMeters><DistanceMeters>9673.861</DistanceMeters><Cadence>76</Cadence><Extensions><TPX xmlns=\"http://www.garmin.com/xmlschemas/ActivityExtension/v2\"><Watts>137</Watts></TPX></Extensions></Trackpoint><Trackpoint><Time>2008-03-03T14:06:29Z</Time><Position><LatitudeDegrees>35.859855</LatitudeDegrees><LongitudeDegrees>-78.886556</LongitudeDegrees></Position><AltitudeMeters>94.347</AltitudeMeters><DistanceMeters>9682.040</DistanceMeters><Cadence>75</Cadence><Extensions><TPX xmlns=\"http://www.garmin.com/xmlschemas/ActivityExtension/v2\"><Watts>138</Watts></TPX></Extensions></Trackpoint><Trackpoint><Time>2008-03-03T14:06:30Z</Time><Position><LatitudeDegrees>35.859838</LatitudeDegrees><LongitudeDegrees>-78.886469</LongitudeDegrees></Position><AltitudeMeters>94.347</AltitudeMeters><DistanceMeters>9690.165</DistanceMeters><Cadence>75</Cadence><Extensions><TPX xmlns=\"http://www.garmin.com/xmlschemas/ActivityExtension/v2\"><Watts>157</Watts></TPX></Extensions></Trackpoint><Trackpoint><Time>2008-03-03T14:06:31Z</Time><Position><LatitudeDegrees>35.859828</LatitudeDegrees><LongitudeDegrees>-78.886380</LongitudeDegrees></Position><AltitudeMeters>94.347</AltitudeMeters><DistanceMeters>9698.242</DistanceMeters><Cadence>75</Cadence><Extensions><TPX xmlns=\"http://www.garmin.com/xmlschemas/ActivityExtension/v2\"><Watts>158</Watts></TPX></Extensions></Trackpoint><Trackpoint><Time>2008-03-03T14:06:32Z</Time><Position><LatitudeDegrees>35.859831</LatitudeDegrees><LongitudeDegrees>-78.886292</LongitudeDegrees></Position><AltitudeMeters>94.827</AltitudeMeters><DistanceMeters>9706.209</DistanceMeters><Cadence>75</Cadence><Extensions><TPX xmlns=\"http://www.garmin.com/xmlschemas/ActivityExtension/v2\"><Watts>166</Watts></TPX></Extensions></Trackpoint><Trackpoint><Time>2008-03-03T14:06:33Z</Time><Position><LatitudeDegrees>35.859850</LatitudeDegrees><LongitudeDegrees>-78.886208</LongitudeDegrees></Position><AltitudeMeters>94.827</AltitudeMeters><DistanceMeters>9714.009</DistanceMeters><Cadence>73</Cadence><Extensions><TPX xmlns=\"http://www.garmin.com/xmlschemas/ActivityExtension/v2\"><Watts>179</Watts></TPX></Extensions></Trackpoint><Trackpoint><Time>2008-03-03T14:06:34Z</Time><Position><LatitudeDegrees>35.859882</LatitudeDegrees><LongitudeDegrees>-78.886132</LongitudeDegrees></Position><AltitudeMeters>95.308</AltitudeMeters><DistanceMeters>9721.714</DistanceMeters><Cadence>73</Cadence><Extensions><TPX xmlns=\"http://www.garmin.com/xmlschemas/ActivityExtension/v2\"><Watts>177</Watts></TPX></Extensions></Trackpoint><Trackpoint><Time>2008-03-03T14:06:35Z</Time><Position><LatitudeDegrees>35.859923</LatitudeDegrees><LongitudeDegrees>-78.886063</LongitudeDegrees></Position><AltitudeMeters>94.827</AltitudeMeters><DistanceMeters>9729.320</DistanceMeters><Cadence>71</Cadence><Extensions><TPX xmlns=\"http://www.garmin.com/xmlschemas/ActivityExtension/v2\"><Watts>184</Watts></TPX></Extensions></Trackpoint><Trackpoint><Time>2008-03-03T14:06:36Z</Time><Position><LatitudeDegrees>35.859972</LatitudeDegrees><LongitudeDegrees>-78.886004</LongitudeDegrees></Position><AltitudeMeters>95.308</AltitudeMeters><DistanceMeters>9736.926</DistanceMeters><Cadence>71</Cadence><Extensions><TPX xmlns=\"http://www.garmin.com/xmlschemas/ActivityExtension/v2\"><Watts>191</Watts></TPX></Extensions></Trackpoint><Trackpoint><Time>2008-03-03T14:06:37Z</Time><Position><LatitudeDegrees>35.860026</LatitudeDegrees><LongitudeDegrees>-78.885953</LongitudeDegrees></Position><AltitudeMeters>94.827</AltitudeMeters><DistanceMeters>9744.549</DistanceMeters><Cadence>71</Cadence><Extensions><TPX xmlns=\"http://www.garmin.com/xmlschemas/ActivityExtension/v2\"><Watts>192</Watts></TPX></Extensions></Trackpoint><Trackpoint><Time>2008-03-03T14:06:38Z</Time><Position><LatitudeDegrees>35.860082</LatitudeDegrees><LongitudeDegrees>-78.885906</LongitudeDegrees></Position><AltitudeMeters>95.308</AltitudeMeters><DistanceMeters>9752.051</DistanceMeters><Cadence>69</Cadence><Extensions><TPX xmlns=\"http://www.garmin.com/xmlschemas/ActivityExtension/v2\"><Watts>210</Watts></TPX></Extensions></Trackpoint><Trackpoint><Time>2008-03-03T14:06:39Z</Time><Position><LatitudeDegrees>35.860136</LatitudeDegrees><LongitudeDegrees>-78.885858</LongitudeDegrees></Position><AltitudeMeters>95.308</AltitudeMeters><DistanceMeters>9759.475</DistanceMeters><Cadence>69</Cadence><Extensions><TPX xmlns=\"http://www.garmin.com/xmlschemas/ActivityExtension/v2\"><Watts>220</Watts></TPX></Extensions></Trackpoint><Trackpoint><Time>2008-03-03T14:06:40Z</Time><Position><LatitudeDegrees>35.860191</LatitudeDegrees><LongitudeDegrees>-78.885809</LongitudeDegrees></Position><AltitudeMeters>95.788</AltitudeMeters><DistanceMeters>9766.951</DistanceMeters><Cadence>69</Cadence><Extensions><TPX xmlns=\"http://www.garmin.com/xmlschemas/ActivityExtension/v2\"><Watts>242</Watts></TPX></Extensions></Trackpoint><Trackpoint><Time>2008-03-03T14:06:41Z</Time><Position><LatitudeDegrees>35.860246</LatitudeDegrees><LongitudeDegrees>-78.885760</LongitudeDegrees></Position><AltitudeMeters>95.788</AltitudeMeters><DistanceMeters>9774.520</DistanceMeters><Cadence>70</Cadence><Extensions><TPX xmlns=\"http://www.garmin.com/xmlschemas/ActivityExtension/v2\"><Watts>280</Watts></TPX></Extensions></Trackpoint><Trackpoint><Time>2008-03-03T14:06:42Z</Time><Position><LatitudeDegrees>35.860301</LatitudeDegrees><LongitudeDegrees>-78.885710</LongitudeDegrees></Position><AltitudeMeters>95.788</AltitudeMeters><DistanceMeters>9782.168</DistanceMeters><Cadence>71</Cadence><Extensions><TPX xmlns=\"http://www.garmin.com/xmlschemas/ActivityExtension/v2\"><Watts>284</Watts></TPX></Extensions></Trackpoint><Trackpoint><Time>2008-03-03T14:06:43Z</Time><Position><LatitudeDegrees>35.860357</LatitudeDegrees><LongitudeDegrees>-78.885660</LongitudeDegrees></Position><AltitudeMeters>95.788</AltitudeMet
